vi "poly_control_signalling_write_self_multi_1.vi"(6 "mode (Sgnl)":T1(ring)=enum."Val(Sgnl)", 8 "error in (no error)":errorcluster, 9 "values":variant[](array[variant]), 10 "control names":string[](array[string])) -> (0 "error out":errorcluster, 2 "control refs":refnum<vi>[](array[refnum]), 4 "found?":bool[](array[boolean]))   [LabVIEW 2015]
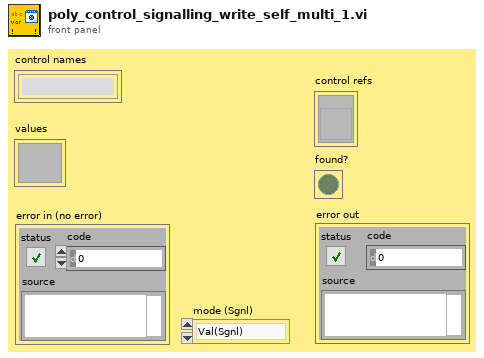
[diagram p1: front panel]
types:
  T1 = enum16{"Val", "Val(Sgnl)", "Val(Undo)", "Method"}
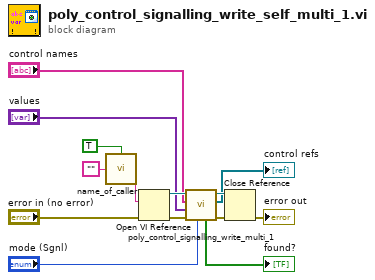
[diagram p0: block diagram]
diagram:
  n1 = call "name_of_caller.vi"("is in inlined vi? (F)"=TRUE, "name of caller in"="") -> ("name of caller out"=w13:string)  [unwired: 2 in]
  n2 = Open VI Reference(vi path=w13, error in (no error)="error in (no error)") -> (vi reference=w12:refnum<vi>, error out=w10:errorcluster)  [unwired: 4 in]
  n3 = call "poly_control_signalling_write_multi_1.vi"("mode (Sgnl)"="mode (Sgnl)", "error in (no error)"=w10, "values"="values", "control names"="control names", "vi reference"=w12) -> ("error out"=w9:errorcluster, "control refs"=→"control refs":refnum<vi>[], "vi reference out"=w11:refnum<vi>, "found?"=→"found?":bool[])  [unwired: 3 in]
  n4 = Close Reference(reference=w11, error in (no error)=w9) -> (error out=→"error out":errorcluster)
